vi "SECADO_JKI_v120.vi"() -> ()   [LabVIEW 2017] (continued)
C"=0.0, "P116.temperatura, C"=0.0, "P116.output, %"=0.0, "P116.output, W"=0.0, "Q.set.caudal, g/s"=0.0, "Q.caudal, g/s"=0.0, "Agua.evapor, g/s"=0.0, "Humedad.lecho, f1"=0.0, "Q.aire.seco, W"=0.0, "Q.evaporacion, W"=0.0, "Porosidad, "=0.0, "Vel.air.reactor, m/s"=0.0, "Temp.termopar.7, C"=0.0, "Temp.termopar.8, C"=0.0, "Temp.termopar.9, C"=0.0, "Presion.abs.ext, Pa"=0.0}, {"Tiempo (min)"=0.0, "Temperatura.ext, C"=0.0, "Humedad.Rel.ext, f1"=0.0, "Temp.pt100.1, C"=0.0, "Temp.pt100.2, C"=0.0, "Temp.pt100.3, C"=0.0, "Temp.pt100.4, C"=0.0, "Temp.termopar.5, C"=0.0, "Temp.termopar.6, C"=0.0, "Humedad.rel.3, f1"=0.0, "Humedad.rel.4, f1"=0.0, "Q.caudal.vol, m3/h"=0.0, "P116.set.temp, C"=0.0, "P116.temperatura, C"=0.0, "P116.output, %"=0.0, "P116.output, W"=0.0, "Q.set.caudal, g/s"=0.0, "Q.caudal, g/s"=0.0, "Agua.evapor, g/s"=0.0, "Humedad.lecho, f1"=0.0, "Q.aire.seco, W"=0.0, "Q.evaporacion, W"=0.0, "Porosidad, "=0.0, "Vel.air.reactor, m/s"=0.0, "Temp.termopar.7, C"=0.0, "Temp.termopar.8, C"=0.0, "Temp.termopar.9, C"=0.0, "Presion.abs.ext, Pa"=0.0}, {"Tiempo (min)"=0.0, "Temperatura.ext, C"=0.0, "Humedad.Rel.ext, f1"=0.0, "Temp.pt100.1, C"=0.0, "Temp.pt100.2, C"=0.0, "Temp.pt100.3, C"=0.0, "Temp.pt100.4, C"=0.0, "Temp.termopar.5, C"=0.0, "Temp.termopar.6, C"=0.0, "Humedad.rel.3, f1"=0.0, "Humedad.rel.4, f1"=0.0, "Q.caudal.vol, m3/h"=0.0, "P116.set.temp, C"=0.0, "P116.temperatura, C"=0.0, "P116.output, %"=0.0, "P116.output, W"=0.0, "Q.set.caudal, g/s"=0.0, "Q.caudal, g/s"=0.0, "Agua.evapor, g/s"=0.0, "Humedad.lecho, f1"=0.0, "Q.aire.seco, W"=0.0, "Q.evaporacion, W"=0.0, "Porosidad, "=0.0, "Vel.air.reactor, m/s"=0.0, "Temp.termopar.7, C"=0.0, "Temp.termopar.8, C"=0.0, "Temp.termopar.9, C"=0.0, "Presion.abs.ext, Pa"=0.0}, {"Tiempo (min)"=0.0, "Temperatura.ext, C"=0.0, "Humedad.Rel.ext, f1"=0.0, "Temp.pt100.1, C"=0.0, "Temp.pt100.2, C"=0.0, "Temp.pt100.3, C"=0.0, "Temp.pt100.4, C"=0.0, "Temp.termopar.5, C"=0.0, "Temp.termopar.6, C"=0.0, "Humedad.rel.3, f1"=0.0, "Humedad.rel.4, f1"=0.0, "Q.caudal.vol, m3/h"=0.0, "P116.set.temp, C"=0.0, "P116.temperatura, C"=0.0, "P116.output, %"=0.0, "P116.output, W"=0.0, "Q.set.caudal, g/s"=0.0, "Q.caudal, g/s"=0.0, "Agua.evapor, g/s"=0.0, "Humedad.lecho, f1"=0.0, "Q.aire.seco, W"=0.0, "Q.evaporacion, W"=0.0, "Porosidad, "=0.0, "Vel.air.reactor, m/s"=0.0, "Temp.termopar.7, C"=0.0, "Temp.termopar.8, C"=0.0, "Temp.termopar.9, C"=0.0, "Presion.abs.ext, Pa"=0.0}, {"Tiempo (min)"=0.0, "Temperatura.ext, C"=0.0, "Humedad.Rel.ext, f1"=0.0, "Temp.pt100.1, C"=0.0, "Temp.pt100.2, C"=0.0, "Temp.pt100.3, C"=0.0, "Temp.pt100.4, C"=0.0, "Temp.termopar.5, C"=0.0, "Temp.termopar.6, C"=0.0, "Humedad.rel.3, f1"=0.0, "Humedad.rel.4, f1"=0.0, "Q.caudal.vol, m3/h"=0.0, "P116.set.temp, C"=0.0, "P116.temperatura, C"=0.0, "P116.output, %"=0.0, "P116.output, W"=0.0, "Q.set.caudal, g/s"=0.0, "Q.caudal, g/s"=0.0, "Agua.evapor, g/s"=0.0, "Humedad.lecho, f1"=0.0, "Q.aire.seco, W"=0.0, "Q.evaporacion, W"=0.0, "Porosidad, "=0.0, "Vel.air.reactor, m/s"=0.0, "Temp.termopar.7, C"=0.0, "Temp.termopar.8, C"=0.0, "Temp.termopar.9, C"=0.0, "Presion.abs.ext, Pa"=0.0}, {"Tiempo (min)"=0.0, "Temperatura.ext, C"=0.0, "Humedad.Rel.ext, f1"=0.0, "Temp.pt100.1, C"=0.0, "Temp.pt100.2, C"=0.0, "Temp.pt100.3, C"=0.0, "Temp.pt100.4, C"=0.0, "Temp.termopar.5, C"=0.0, "Temp.termopar.6, C"=0.0, "Humedad.rel.3, f1"=0.0, "Humedad.rel.4, f1"=0.0, "Q.caudal.vol, m3/h"=0.0, "P116.set.temp, C"=0.0, "P116.temperatura, C"=0.0, "P116.output, %"=0.0, "P116.output, W"=0.0, "Q.set.caudal, g/s"=0.0, "Q.caudal, g/s"=0.0, "Agua.evapor, g/s"=0.0, "Humedad.lecho, f1"=0.0, "Q.aire.seco, W"=0.0, "Q.evaporacion, W"=0.0, "Porosidad, "=0.0, "Vel.air.reactor, m/s"=0.0, "Temp.termopar.7, C"=0.0, "Temp.termopar.8, C"=0.0, "Temp.termopar.9, C"=0.0, "Presion.abs.ext, Pa"=0.0}, {"Tiempo (min)"=0.0, "Temperatura.ext, C"=0.0, "Humedad.Rel.ext, f1"=0.0, "Temp.pt100.1, C"=0.0, "Temp.pt100.2, C"=0.0, "Temp.pt100.3, C"=0.0, "Temp.pt100.4, C"=0.0, "Temp.termopar.5, C"=0.0, "Temp.termopar.6, C"=0.0, "Humedad.rel.3, f1"=0.0, "Humedad.rel.4, f1"=0.0, "Q.caudal.vol, m3/h"=0.0, "P116.set.temp, C"=0.0, "P116.temperatura, C"=0.0, "P116.output, %"=0.0, "P116.output, W"=0.0, "Q.set.caudal, g/s"=0.0, "Q.caudal, g/s"=0.0, "Agua.evapor, g/s"=0.0, "Humedad.lecho, f1"=0.0, "Q.aire.seco, W"=0.0, "Q.evaporacion, W"=0.0, "Porosidad, "=0.0, "Vel.air.reactor, m/s"=0.0, "Temp.termopar.7, C"=0.0, "Temp.termopar.8, C"=0.0, "Temp.termopar.9, C"=0.0, "Presion.abs.ext, Pa"=0.0}, {"Tiempo (min)"=0.0, "Temperatura.ext, C"=0.0, "Humedad.Rel.ext, f1"=0.0, "Temp.pt100.1, C"=0.0, "Temp.pt100.2, C"=0.0, "Temp.pt100.3, C"=0.0, "Temp.pt100.4, C"=0.0, "Temp.termopar.5, C"=0.0, "Temp.termopar.6, C"=0.0, "Humedad.rel.3, f1"=0.0, "Humedad.rel.4, f1"=0.0, "Q.caudal.vol, m3/h"=0.0, "P116.set.temp, C"=0.0, "P116.temperatura, C"=0.0, "P116.output, %"=0.0, "P116.output, W"=0.0, "Q.set.caudal, g/s"=0.0, "Q.caudal, g/s"=0.0, "Agua.evapor, g/s"=0.0, "Humedad.lecho, f1"=0.0, "Q.aire.seco, W"=0.0, "Q.evaporacion, W"=0.0, "Porosidad, "=0.0, "Vel.air.reactor, m/s"=0.0, "Temp.termopar.7, C"=0.0, "Temp.termopar.8, C"=0.0, "Temp.termopar.9, C"=0.0, "Presion.abs.ext, Pa"=0.0}, {"Tiempo (min)"=0.0, "Temperatura.ext, C"=0.0, "Humedad.Rel.ext, f1"=0.0, "Temp.pt100.1, C"=0.0, "Temp.pt100.2, C"=0.0, "Temp.pt100.3, C"=0.0, "Temp.pt100.4, C"=0.0, "Temp.termopar.5, C"=0.0, "Temp.termopar.6, C"=0.0, "Humedad.rel.3, f1"=0.0, "Humedad.rel.4, f1"=0.0, "Q.caudal.vol, m3/h"=0.0, "P116.set.temp, C"=0.0, "P116.temperatura, C"=0.0, "P116.output, %"=0.0, "P116.output, W"=0.0, "Q.set.caudal, g/s"=0.0, "Q.caudal, g/s"=0.0, "Agua.evapor, g/s"=0.0, "Humedad.lecho, f1"=0.0, "Q.aire.seco, W"=0.0, "Q.evaporacion, W"=0.0, "Porosidad, "=0.0, "Vel.air.reactor, m/s"=0.0, "Temp.termopar.7, C"=0.0, "Temp.termopar.8, C"=0.0, "Temp.termopar.9, C"=0.0, "Presion.abs.ext, Pa"=0.0}, {"Tiempo (min)"=0.0, "Temperatura.ext, C"=0.0, "Humedad.Rel.ext, f1"=0.0, "Temp.pt100.1, C"=0.0, "Temp.pt100.2, C"=0.0, "Temp.pt100.3, C"=0.0, "Temp.pt100.4, C"=0.0, "Temp.termopar.5, C"=0.0, "Temp.termopar.6, C"=0.0, "Humedad.rel.3, f1"=0.0, "Humedad.rel.4, f1"=0.0, "Q.caudal.vol, m3/h"=0.0, "P116.set.temp, C"=0.0, "P116.temperatura, C"=0.0, "P116.output, %"=0.0, "P116.output, W"=0.0, "Q.set.caudal, g/s"=0.0, "Q.caudal, g/s"=0.0, "Agua.evapor, g/s"=0.0, "Humedad.lecho, f1"=0.0, "Q.aire.seco, W"=0.0, "Q.evaporacion, W"=0.0, "Porosidad, "=0.0, "Vel.air.reactor, m/s"=0.0, "Temp.termopar.7, C"=0.0, "Temp.termopar.8, C"=0.0, "Temp.termopar.9, C"=0.0, "Presion.abs.ext, Pa"=0.0}, {"Tiempo (min)"=0.0, "Temperatura.ext, C"=0.0, "Humedad.Rel.ext, f1"=0.0, "Temp.pt100.1, C"=0.0, "Temp.pt100.2, C"=0.0, "Temp.pt100.3, C"=0.0, "Temp.pt100.4, C"=0.0, "Temp.termopar.5, C"=0.0, "Temp.termopar.6, C"=0.0, "Humedad.rel.3, f1"=0.0, "Humedad.rel.4, f1"=0.0, "Q.caudal.vol, m3/h"=0.0, "P116.set.temp, C"=0.0, "P116.temperatura, C"=0.0, "P116.output, %"=0.0, "P116.output, W"=0.0, "Q.set.caudal, g/s"=0.0, "Q.caudal, g/s"=0.0, "Agua.evapor, g/s"=0.0, "Humedad.lecho, f1"=0.0, "Q.aire.seco, W"=0.0, "Q.evaporacion, W"=0.0, "Porosidad, "=0.0, "Vel.air.reactor, m/s"=0.0, "Temp.termopar.7, C"=0.0, "Temp.termopar.8, C"=0.0, "Temp.termopar.9, C"=0.0, "Presion.abs.ext, Pa"=0.0}, {"Tiempo (min)"=0.0, "Temperatura.ext, C"=0.0, "Humedad.Rel.ext, f1"=0.0, "Temp.pt100.1, C"=0.0, "Temp.pt100.2, C"=0.0, "Temp.pt100.3, C"=0.0, "Temp.pt100.4, C"=0.0, "Temp.termopar.5, C"=0.0, "Temp.termopar.6, C"=0.0, "Humedad.rel.3, f1"=0.0, "Humedad.rel.4, f1"=0.0, "Q.caudal.vol, m3/h"=0.0, "P116.set.temp, C"=0.0, "P116.temperatura, C"=0.0, "P116.output, %"=0.0, "P116.output, W"=0.0, "Q.set.caudal, g/s"=0.0, "Q.caudal, g/s"=0.0, "Agua.evapor, g/s"=0.0, "Humedad.lecho, f1"=0.0, "Q.aire.seco, W"=0.0, "Q.evaporacion, W"=0.0, "Porosidad, "=0.0, "Vel.air.reactor, m/s"=0.0, "Temp.termopar.7, C"=0.0, "Temp.termopar.8, C"=0.0, "Temp.termopar.9, C"=0.0, "Presion.abs.ext, Pa"=0.0}, {"Tiempo (min)"=0.0, "Temperatura.ext, C"=0.0, "Humedad.Rel.ext, f1"=0.0, "Temp.pt100.1, C"=0.0, "Temp.pt100.2, C"=0.0, "Temp.pt100.3, C"=0.0, "Temp.pt100.4, C"=0.0, "Temp.termopar.5, C"=0.0, "Temp.termopar.6, C"=0.0, "Humedad.rel.3, f1"=0.0, "Humedad.rel.4, f1"=0.0, "Q.caudal.vol, m3/h"=0.0, "P116.set.temp, C"=0.0, "P116.temperatura, C"=0.0, "P116.output, %"=0.0, "P116.output, W"=0.0, "Q.set.caudal, g/s"=0.0, "Q.caudal, g/s"=0.0, "Agua.evapor, g/s"=0.0, "Humedad.lecho, f1"=0.0, "Q.aire.seco, W"=0.0, "Q.evaporacion, W"=0.0, "Porosidad, "=0.0, "Vel.air.reactor, m/s"=0.0, "Temp.termopar.7, C"=0.0, "Temp.termopar.8, C"=0.0, "Temp.termopar.9, C"=0.0, "Presion.abs.ext, Pa"=0.0}, {"Tiempo (min)"=0.0, "Temperatura.ext, C"=0.0, "Humedad.Rel.ext, f1"=0.0, "Temp.pt100.1, C"=0.0, "Temp.pt100.2, C"=0.0, "Temp.pt100.3, C"=0.0, "Temp.pt100.4, C"=0.0, "Temp.termopar.5, C"=0.0, "Temp.termopar.6, C"=0.0, "Humedad.rel.3, f1"=0.0, "Humedad.rel.4, f1"=0.0, "Q.caudal.vol, m3/h"=0.0, "P116.set.temp, C"=0.0, "P116.temperatura, C"=0.0, "P116.output, %"=0.0, "P116.output, W"=0.0, "Q.set.caudal, g/s"=0.0, "Q.caudal, g/s"=0.0, "Agua.evapor, g/s"=0.0, "Humedad.lecho, f1"=0.0, "Q.aire.seco, W"=0.0, "Q.evaporacion, W"=0.0, "Porosidad, "=0.0, "Vel.air.reactor, m/s"=0.0, "Temp.termopar.7, C"=0.0, "Temp.termopar.8, C"=0.0, "Temp.termopar.9, C"=0.0, "Presion.abs.ext, Pa"=0.0}, {"Tiempo (min)"=0.0, "Temperatura.ext, C"=0.0, "Humedad.Rel.ext, f1"=0.0, "Temp.pt100.1, C"=0.0, "Temp.pt100.2, C"=0.0, "Temp.pt100.3, C"=0.0, "Temp.pt100.4, C"=0.0, "Temp.termopar.5, C"=0.0, "Temp.termopar.6, C"=0.0, "Humedad.rel.3, f1"=0.0, "Humedad.rel.4, f1"=0.0, "Q.caudal.vol, m3/h"=0.0, "P116.set.temp, C"=0.0, "P116.temperatura, C"=0.0, "P116.output, %"=0.0, "P116.output, W"=0.0, "Q.set.caudal, g/s"=0.0, "Q.caudal, g/s"=0.0, "Agua.evapor, g/s"=0.0, "Humedad.lecho, f1"=0.0, "Q.aire.seco, W"=0.0, "Q.evaporacion, W"=0.0, "Porosidad, "=0.0, "Vel.air.reactor, m/s"=0.0, "Temp.termopar.7, C"=0.0, "Temp.termopar.8, C"=0.0, "Temp.termopar.9, C"=0.0, "Presion.abs.ext, Pa"=0.0}, {"Tiempo (min)"=0.0, "Temperatura.ext, C"=0.0, "Humedad.Rel.ext, f1"=0.0, "Temp.pt100.1, C"=0.0, "Temp.pt100.2, C"=0.0, "Temp.pt100.3, C"=0.0, "Temp.pt100.4, C"=0.0, "Temp.termopar.5, C"=0.0, "Temp.termopar.6, C"=0.0, "Humedad.rel.3, f1"=0.0, "Humedad.rel.4, f1"=0.0, "Q.caudal.vol, m3/h"=0.0, "P116.set.temp, C"=0.0, "P116.temperatura, C"=0.0, "P116.output, %"=0.0, "P116.output, W"=0.0, "Q.set.caudal, g/s"=0.0, "Q.caudal, g/s"=0.0, "Agua.evapor, g/s"=0.0, "Humedad.lecho, f1"=0.0, "Q.aire.seco, W"=0.0, "Q.evaporacion, W"=0.0, "Porosidad, "=0.0, "Vel.air.reactor, m/s"=0.0, "Temp.termopar.7, C"=0.0, "Temp.termopar.8, C"=0.0, "Temp.termopar.9, C"=0.0, "Presion.abs.ext, Pa"=0.0}, {"Tiempo (min)"=0.0, "Temperatura.ext, C"=0.0, "Humedad.Rel.ext, f1"=0.0, "Temp.pt100.1, C"=0.0, "Temp.pt100.2, C"=0.0, "Temp.pt100.3, C"=0.0, "Temp.pt100.4, C"=0.0, "Temp.termopar.5, C"=0.0, "Temp.termopar.6, C"=0.0, "Humedad.rel.3, f1"=0.0, "Humedad.rel.4, f1"=0.0, "Q.caudal.vol, m3/h"=0.0, "P116.set.temp, C"=0.0, "P116.temperatura, C"=0.0, "P116.output, %"=0.0, "P116.output, W"=0.0, "Q.set.caudal, g/s"=0.0, "Q.caudal, g/s"=0.0, "Agua.evapor, g/s"=0.0, "Humedad.lecho, f1"=0.0, "Q.aire.seco, W"=0.0, "Q.evaporacion, W"=0.0, "Porosidad, "=0.0, "Vel.air.reactor, m/s"=0.0, "Temp.termopar.7, C"=0.0, "Temp.termopar.8, C"=0.0, "Temp.termopar.9, C"=0.0, "Presion.abs.ext, Pa"=0.0}, {"Tiempo (min)"=0.0, "Temperatura.ext, C"=0.0, "Humedad.Rel.ext, f1"=0.0, "Temp.pt100.1, C"=0.0, "Temp.pt100.2, C"=0.0, "Temp.pt100.3, C"=0.0, "Temp.pt100.4, C"=0.0, "Temp.termopar.5, C"=0.0, "Temp.termopar.6, C"=0.0, "Humedad.rel.3, f1"=0.0, "Humedad.rel.4, f1"=0.0, "Q.caudal.vol, m3/h"=0.0, "P116.set.temp, C"=0.0, "P116.temperatura, C"=0.0, "P116.output, %"=0.0, "P116.output, W"=0.0, "Q.set.caudal, g/s"=0.0, "Q.caudal, g/s"=0.0, "Agua.evapor, g/s"=0.0, "Humedad.lecho, f1"=0.0, "Q.aire.seco, W"=0.0, "Q.evaporacion, W"=0.0, "Porosidad, "=0.0, "Vel.air.reactor, m/s"=0.0, "Temp.termopar.7, C"=0.0, "Temp.termopar.8, C"=0.0, "Temp.termopar.9, C"=0.0, "Presion.abs.ext, Pa"=0.0}, {"Tiempo (min)"=0.0, "Temperatura.ext, C"=0.0, "Humedad.Rel.ext, f1"=0.0, "Temp.pt100.1, C"=0.0, "Temp.pt100.2, C"=0.0, "Temp.pt100.3, C"=0.0, "Temp.pt100.4, C"=0.0, "Temp.termopar.5, C"=0.0, "Temp.termopar.6, C"=0.0, "Humedad.rel.3, f1"=0.0, "Humedad.rel.4, f1"=0.0, "Q.caudal.vol, m3/h"=0.0, "P116.set.temp, C"=0.0, "P116.temperatura, C"=0.0, "P116.output, %"=0.0, "P116.output, W"=0.0, "Q.set.caudal, g/s"=0.0, "Q.caudal, g/s"=0.0, "Agua.evapor, g/s"=0.0, "Humedad.lecho, f1"=0.0, "Q.aire.seco, W"=0.0, "Q.evaporacion, W"=0.0, "Porosidad, "=0.0, "Vel.air.reactor, m/s"=0.0, "Temp.termopar.7, C"=0.0, "Temp.termopar.8, C"=0.0, "Temp.termopar.9, C"=0.0, "Presion.abs.ext, Pa"=0.0}, {"Tiempo (min)"=0.0, "Temperatura.ext, C"=0.0, "Humedad.Rel.ext, f1"=0.0, "Temp.pt100.1, C"=0.0, "Temp.pt100.2, C"=0.0, "Temp.pt100.3, C"=0.0, "Temp.pt100.4, C"=0.0, "Temp.termopar.5, C"=0.0, "Temp.termopar.6, C"=0.0, "Humedad.rel.3, f1"=0.0, "Humedad.rel.4, f1"=0.0, "Q.caudal.vol, m3/h"=0.0, "P116.set.temp, C"=0.0, "P116.temperatura, C"=0.0, "P116.output, %"=0.0, "P116.output, W"=0.0, "Q.set.caudal, g/s"=0.0, "Q.caudal, g/s"=0.0, "Agua.evapor, g/s"=0.0, "Humedad.lecho, f1"=0.0, "Q.aire.seco, W"=0.0, "Q.evaporacion, W"=0.0, "Porosidad, "=0.0, "Vel.air.reactor, m/s"=0.0, "Temp.termopar.7, C"=0.0, "Temp.termopar.8, C"=0.0, "Temp.termopar.9, C"=0.0, "Presion.abs.ext, Pa"=0.0}, {"Tiempo (min)"=0.0, "Temperatura.ext, C"=0.0, "Humedad.Rel.ext, f1"=0.0, "Temp.pt100.1, C"=0.0, "Temp.pt100.2, C"=0.0, "Temp.pt100.3, C"=0.0, "Temp.pt100.4, C"=0.0, "Temp.termopar.5, C"=0.0, "Temp.termopar.6, C"=0.0, "Humedad.rel.3, f1"=0.0, "Humedad.rel.4, f1"=0.0, "Q.caudal.vol, m3/h"=0.0, "P116.set.temp, C"=0.0, "P116.temperatura, C"=0.0, "P116.output, %"=0.0, "P116.output, W"=0.0, "Q.set.caudal, g/s"=0.0, "Q.caudal, g/s"=0.0, "Agua.evapor, g/s"=0.0, "Humedad.lecho, f1"=0.0, "Q.aire.seco, W"=0.0, "Q.evaporacion, W"=0.0, "Porosidad, "=0.0, "Vel.air.reactor, m/s"=0.0, "Temp.termopar.7, C"=0.0, "Temp.termopar.8, C"=0.0, "Temp.termopar.9, C"=0.0, "Presion.abs.ext, Pa"=0.0}, {"Tiempo (min)"=0.0, "Temperatura.ext, C"=0.0, "Humedad.Rel.ext, f1"=0.0, "Temp.pt100.1, C"=0.0, "Temp.pt100.2, C"=0.0, "Temp.pt100.3, C"=0.0, "Temp.pt100.4, C"=0.0, "Temp.termopar.5, C"=0.0, "Temp.termopar.6, C"=0.0, "Humedad.rel.3, f1"=0.0, "Humedad.rel.4, f1"=0.0, "Q.caudal.vol, m3/h"=0.0, "P116.set.temp, C"=0.0, "P116.temperatura, C"=0.0, "P116.output, %"=0.0, "P116.output, W"=0.0, "Q.set.caudal, g/s"=0.0, "Q.caudal, g/s"=0.0, "Agua.evapor, g/s"=0.0, "Humedad.lecho, f1"=0.0, "Q.aire.seco, W"=0.0, "Q.evaporacion, W"=0.0, "Porosidad, "=0.0, "Vel.air.reactor, m/s"=0.0, "Temp.termopar.7, C"=0.0, "Temp.termopar.8, C"=0.0, "Temp.termopar.9, C"=0.0, "Presion.abs.ext, Pa"=0.0}, {"Tiempo (min)"=0.0, "Temperatura.ext, C"=0.0, "Humedad.Rel.ext, f1"=0.0, "Temp.pt100.1, C"=0.0, "Temp.pt100.2, C"=0.0, "Temp.pt100.3, C"=0.0, "Temp.pt100.4, C"=0.0, "Temp.termopar.5, C"=0.0, "Temp.termopar.6, C"=0.0, "Humedad.rel.3, f1"=0.0, "Humedad.rel.4, f1"=0.0, "Q.caudal.vol, m3/h"=0.0, "P116.set.temp, C"=0.0, "P116.temperatura, C"=0.0, "P116.output, %"=0.0, "P116.output, W"=0.0, "Q.set.caudal, g/s"=0.0, "Q.caudal, g/s"=0.0, "Agua.evapor, g/s"=0.0, "Humedad.lecho, f1"=0.0, "Q.aire.seco, W"=0.0, "Q.evaporacion, W"=0.0, "Porosidad, "=0.0, "Vel.air.reactor, m/s"=0.0, "Temp.termopar.7, C"=0.0, "Temp.termopar.8, C"=0.0, "Temp.termopar.9, C"=0.0, "Presion.abs.ext, Pa"=0.0}, {"Tiempo (min)"=0.0, "Temperatura.ext, C"=0.0, "Humedad.Rel.ext, f1"=0.0, "Temp.pt100.1, C"=0.0, "Temp.pt100.2, C"=0.0, "Temp.pt100.3, C"=0.0, "Temp.pt100.4, C"=0.0, "Temp.termopar.5, C"=0.0, "Temp.termopar.6, C"=0.0, "Humedad.rel.3, f1"=0.0, "Humedad.rel.4, f1"=0.0, "Q.caudal.vol, m3/h"=0.0, "P116.set.temp, C"=0.0, "P116.temperatura, C"=0.0, "P116.output, %"=0.0, "P116.output, W"=0.0, "Q.set.caudal, g/s"=0.0, "Q.caudal, g/s"=0.0, "Agua.evapor, g/s"=0.0, "Humedad.lecho, f1"=0.0, "Q.aire.seco, W"=0.0, "Q.evaporacion, W"=0.0, "Porosidad, "=0.0, "Vel.air.reactor, m/s"=0.0, "Temp.termopar.7, C"=0.0, "Temp.termopar.8, C"=0.0, "Temp.termopar.9, C"=0.0, "Presion.abs.ext, Pa"=0.0}, {"Tiempo (min)"=0.0, "Temperatura.ext, C"=0.0, "Humedad.Rel.ext, f1"=0.0, "Temp.pt100.1, C"=0.0, "Temp.pt100.2, C"=0.0, "Temp.pt100.3, C"=0.0, "Temp.pt100.4, C"=0.0, "Temp.termopar.5, C"=0.0, "Temp.termopar.6, C"=0.0, "Humedad.rel.3, f1"=0.0, "Humedad.rel.4, f1"=0.0, "Q.caudal.vol, m3/h"=0.0, "P116.set.temp, C"=0.0, "P116.temperatura, C"=0.0, "P116.output, %"=0.0, "P116.output, W"=0.0, "Q.set.caudal, g/s"=0.0, "Q.caudal, g/s"=0.0, "Agua.evapor, g/s"=0.0, "Humedad.lecho, f1"=0.0, "Q.aire.seco, W"=0.0, "Q.evaporacion, W"=0.0, "Porosidad, "=0.0, "Vel.air.reactor, m/s"=0.0, "Temp.termopar.7, C"=0.0, "Temp.termopar.8, C"=0.0, "Temp.termopar.9, C"=0.0, "Presion.abs.ext, Pa"=0.0}, {"Tiempo (min)"=0.0, "Temperatura.ext, C"=0.0, "Humedad.Rel.ext, f1"=0.0, "Temp.pt100.1, C"=0.0, "Temp.pt100.2, C"=0.0, "Temp.pt100.3, C"=0.0, "Temp.pt100.4, C"=0.0, "Temp.termopar.5, C"=0.0, "Temp.termopar.6, C"=0.0, "Humedad.rel.3, f1"=0.0, "Humedad.rel.4, f1"=0.0, "Q.caudal.vol, m3/h"=0.0, "P116.set.temp, C"=0.0, "P116.temperatura, C"=0.0, "P116.output, %"=0.0, "P116.output, W"=0.0, "Q.set.caudal, g/s"=0.0, "Q.caudal, g/s"=0.0, "Agua.evapor, g/s"=0.0, "Humedad.lecho, f1"=0.0, "Q.aire.seco, W"=0.0, "Q.evaporacion, W"=0.0, "Porosidad, "=0.0, "Vel.air.reactor, m/s"=0.0, "Temp.termopar.7, C"=0.0, "Temp.termopar.8, C"=0.0, "Temp.termopar.9, C"=0.0, "Presion.abs.ext, Pa"=0.0}, {"Tiempo (min)"=0.0, "Temperatura.ext, C"=0.0, "Humedad.Rel.ext, f1"=0.0, "Temp.pt100.1, C"=0.0, "Temp.pt100.2, C"=0.0, "Temp.pt100.3, C"=0.0, "Temp.pt100.4, C"=0.0, "Temp.termopar.5, C"=0.0, "Temp.termopar.6, C"=0.0, "Humedad.rel.3, f1"=0.0, "Humedad.rel.4, f1"=0.0, "Q.caudal.vol, m3/h"=0.0, "P116.set.temp, C"=0.0, "P116.temperatura, C"=0.0, "P116.output, %"=0.0, "P116.output, W"=0.0, "Q.set.caudal, g/s"=0.0, "Q.caudal, g/s"=0.0, "Agua.evapor, g/s"=0.0, "Humedad.lecho, f1"=0.0, "Q.aire.seco, W"=0.0, "Q.evaporacion, W"=0.0, "Porosidad, "=0.0, "Vel.air.reactor, m/s"=0.0, "Temp.termopar.7, C"=0.0, "Temp.termopar.8, C"=0.0, "Temp.termopar.9, C"=0.0, "Presion.abs.ext, Pa"=0.0}, {"Tiempo (min)"=0.0, "Temperatura.ext, C"=0.0, "Humedad.Rel.ext, f1"=0.0, "Temp.pt100.1, C"=0.0, "Temp.pt100.2, C"=0.0, "Temp.pt100.3, C"=0.0, "Temp.pt100.4, C"=0.0, "Temp.termopar.5, C"=0.0, "Temp.termopar.6, C"=0.0, "Humedad.rel.3, f1"=0.0, "Humedad.rel.4, f1"=0.0, "Q.caudal.vol, m3/h"=0.0, "P116.set.temp, C"=0.0, "P116.temperatura, C"=0.0, "P116.output, %"=0.0, "P116.output, W"=0.0, "Q.set.caudal, g/s"=0.0, "Q.caudal, g/s"=0.0, "Agua.evapor, g/s"=0.0, "Humedad.lecho, f1"=0.0, "Q.aire.seco, W"=0.0, "Q.evaporacion, W"=0.0, "Porosidad, "=0.0, "Vel.air.reactor, m/s"=0.0, "Temp.termopar.7, C"=0.0, "Temp.termopar.8, C"=0.0, "Temp.termopar.9, C"=0.0, "Presion.abs.ext, Pa"=0.0}]  # data array
        w122 = path "C:/Users/usuario/Documents/LabVIEW Data/testSecado.dat"  # Filename
        w125 = FALSE  # Step.timeout?
        w123 = ""  # Status string
        # "Número de datos maximo para graficar"
        # "Array de datos: rellenar constante con 3600 registros a 0"
        # "Initialize the shift-register data, here.\n(data names are defined by what you wire into the bundle function)"
        n39 = Bundle By Name(cluster=w132, "datos.Ensayo"=w129, "data array"=w130, "nPuntos"=w121, "Filename"=w122, "Status.string"=w123, "Step.sample.time"=w124, "Step.timeout?"=w125, "Prog.running?"=w126, "Prog.aborted?"=w127, "Seq.loaded?"=w128, "#Datos"=w120) -> (w131:T19)
        n40 = call <vilib>:"Add State(s) to Queue__JKI_lib_State_Machine.vi"("State(s) in (\"\")"=w135) -> ("States Out"=w134:string)  [unwired: 14 in]
      }
      frame "Data: Cleanup" {
        # "Cleanup any data and references, here.\n(this is called automatically, by the Macro: Exit)"
        n41 = Unbundle By Name(w136) -> ("Core.Current VI Reference"=w139:refnum<vi>)
        n42 = Close Reference(reference=w139, error in (no error)=w138) -> (error out=w137:errorcluster)
        n43 = call <vilib>:"Add State(s) to Queue__JKI_lib_State_Machine.vi"("State(s) in (\"\")"=w141) -> ("States Out"=w140:string)  [unwired: 14 in]
      }
      frame "---------- Instruments ----------" {
        # "Do not put any code in this frame.\n(It is a separator no-op. You can make a copy of this frame to create a new Data frame)"
        n44 = call <vilib>:"Add State(s) to Queue__JKI_lib_State_Machine.vi"("State(s) in (\"\")"=w145) -> ("States Out"=w144:string)  [unwired: 14 in]
      }
      frame "Instruments: Serial Comms" {
        # "Your code here.\n(You can make a copy of, or modify, this frame)"
        n45 = call "SECADO_enterComms.vi"("error in (no error)"=w149) -> ("error out"=w148:errorcluster, "Comunicaciones"=w146:T9)  [unwired: 8 in, 1 out]
        n46 = Bundle By Name(cluster=w150, "Comunicaciones"=w146) -> (w147:T19)
        n47 = call <vilib>:"Add State(s) to Queue__JKI_lib_State_Machine.vi"("State(s) in (\"\")"=w152) -> ("States Out"=w151:string)  [unwired: 14 in]
      }
      frame "Instruments: Agilent Initialize" {
        # "Read Agilent channels\n(only for information)"
        # "Your code here.\n(You can make a copy of, or modify, this frame)"
        n48 = Unbundle By Name(w159) -> ("Comunicaciones.AGL"=w157:bool, "Comunicaciones.Agilent"=w158:refnum<visa-resource-name>)
        n49 = call "Agilent ReadConfigFile.vi"("Error In"=w154) -> ("Error Out"=w153:errorcluster, "Dispositivos"=→"Dispositivos":T3, "configuration file path"=→"Agilent.configuracion.file":path)  [unwired: 7 in]
        n50 = call "34970_Module.vi"("Agilent 34970A"=w157, "Command"=34970_Module_Control."INICIALIZA", "error in (no error)"=w153, "VISA Agilent 34970A"=w158) -> ("error out"=w160:errorcluster)  [unwired: 3 in, 4 out]
        n51 = call <vilib>:"Add State(s) to Queue__JKI_lib_State_Machine.vi"("State(s) in (\"\")"=w163) -> ("States Out"=w162:string)  [unwired: 14 in]
      }
      frame "Instruments: Agilent Close" {
        # "Your code here.\n(You can make a copy of, or modify, this frame)"
        n52 = Unbundle By Name(w167) -> ("Comunicaciones.AGL"=w165:bool, "Comunicaciones.Agilent"=w166:refnum<visa-resource-name>)
        n53 = call "34970_Module.vi"("Agilent 34970A"=w165, "Command"=34970_Module_Control."SHUTDOWN", "error in (no error)"=w164, "VISA Agilent 34970A"=w166) -> ("error out"=w168:errorcluster)  [unwired: 3 in, 4 out]
        n54 = call <vilib>:"Add State(s) to Queue__JKI_lib_State_Machine.vi"("State(s) in (\"\")"=w171) -> ("States Out"=w170:string)  [unwired: 14 in]
      }
      frame "Instruments: Eurotherm Initialize" {
        # "Your code here.\n(Eurotherm se inicializa, lee (o programa) y cierra en la misma ventana)"
        # "Your code here.\n(You can make a copy of, or modify, this frame)"
        n55 = Unbundle By Name(w173) -> ()  [unwired: 3 out]
        n56 = call <vilib>:"Add State(s) to Queue__JKI_lib_State_Machine.vi"("State(s) in (\"\")"=w175) -> ("States Out"=w174:string)  [unwired: 14 in]
      }
      frame "Instruments: Eurotherm Close" {
        # "Your code here.\n(Eurotherm se inicializa, lee (o programa) y cierra en la misma ventana)"
        # "Your code here.\n(You can make a copy of, or modify, this frame)"
        n57 = Unbundle By Name(w177) -> ()  [unwired: 2 out]
        n58 = call <vilib>:"Add State(s) to Queue__JKI_lib_State_Machine.vi"("State(s) in (\"\")"=w179) -> ("States Out"=w178:string)  [unwired: 14 in]
      }
      frame "---------- Timing ----------" {
        # "Do not put any code in this frame.\n(It is a separator no-op. You can make a copy of this frame to create a new UI frame)"
        n59 = call <vilib>:"Add State(s) to Queue__JKI_lib_State_Machine.vi"("State(s) in (\"\")"=w183) -> ("States Out"=w182:string)  [unwired: 14 in]
      }
      frame "Timing: Initialize Total Time" {
        # "Initialize total time counter in minutes here.\n(data names are defined by what you wire into the bundle function)"
        n60 = call "elapsedTotalMinutesModule.vi"("Command"=Timing_Module_Control."Initialize Time", "error in (no error)"=w185) -> ("error out"=w184:errorcluster)  [unwired: 7 in, 2 out]
        n61 = call <vilib>:"Add State(s) to Queue__JKI_lib_State_Machine.vi"("State(s) in (\"\")"=w189) -> ("States Out"=w188:string)  [unwired: 14 in]
      }
      frame "Timing: Measure Total Time" {
        # "Initialize total time counter in minutes here.\n(data names are defined by what you wire into the bundle function)"
        n62 = call "elapsedTotalMinutesModule.vi"("Command"=Timing_Module_Control."Check Time", "error in (no error)"=w198) -> ("error out"=w197:errorcluster, "Elapsed Out"=w192:dbl)  [unwired: 7 in, 1 out]
        n63 = Unbundle By Name(w191) -> ("datos.Ensayo.Tiempo (min)"=w195:dbl)
        n64 = Subtract(x=w192, y=w195) -> (x-y=w194:dbl)
        n65 = Multiply(x=w194, y=60.0) -> (x*y=w190:dbl)
        "dt.ciclo, s" <- w190
        n66 = Bundle By Name(cluster=w191, "datos.Ensayo.Tiempo (min)"=w192, "delta.t.ciclo"=w190) -> (w196:T19)
        n67 = call <vilib>:"Add State(s) to Queue__JKI_lib_State_Machine.vi"("State(s) in (\"\")"=w201) -> ("States Out"=w200:string)  [unwired: 14 in]
      }
      frame "Timing: Initialize Sample Time" {
        # "Initialize sample time in seconds, used for next sample\n(data names are defined by what you wire into the bundle function)"
        n68 = call "elapsedSamplingSecondsModule.vi"("Command"=Timing_Module_Control."Initialize Time", "error in (no error)"=w206) -> ("error out"=w205:errorcluster)  [unwired: 7 in, 2 out]
        n69 = Bundle By Name(cluster=w207, "Step.timeout?"=FALSE ("Step Timeout?")) -> (w203:T19)
        n70 = call <vilib>:"Add State(s) to Queue__JKI_lib_State_Machine.vi"("State(s) in (\"\")"=w209) -> ("States Out"=w208:string)  [unwired: 14 in]
      }
      frame "Timing: Measure Sample Time" {
        # "Initialize total time counter in minutes here.\n(data names are defined by what you wire into the bundle function)"
        n71 = Multiply(x="t.muestreo, s", y=1.0 ("x")) -> (x*y=w215:dbl)
        n72 = call "elapsedSamplingSecondsModule.vi"("Command"=Timing_Module_Control."Check Time", "error in (no error)"=w218, "Time In"=w215) -> ("error out"=w217:errorcluster, "Elapsed Out"=w212:dbl, "Time Elapsed"=w213:bool)  [unwired: 6 in]
        "t.ciclo, s" <- w212
        n73 = Bundle By Name(cluster=w219, "Step.timeout?"=w213, "Step.sample.time"=w212) -> (w214:T19)
        n74 = call <vilib>:"Add State(s) to Queue__JKI_lib_State_Machine.vi"("State(s) in (\"\")"=w221) -> ("States Out"=w220:string)  [unwired: 14 in]
      }
      frame "---------- UI ----------" {
        # "Do not put any code in this frame.\n(It is a separator no-op. You can make a copy of this frame to create a new UI frame)"
        n75 = call <vilib>:"Add State(s) to Queue__JKI_lib_State_Machine.vi"("State(s) in (\"\")"=w225) -> ("States Out"=w224:string)  [unwired: 14 in]
      }
      frame "UI: Initialize" {
        # "Initialize the User Interface, here.\n(this is called automatically, by the Macro: Init)"
        n76 = call <vilib>:"Add State(s) to Queue__JKI_lib_State_Machine.vi"("State(s) in (\"\")"=w229) -> ("States Out"=w228:string)  [unwired: 14 in]
      }
      frame "UI: Cursor Set" {
        # "Argument"
        # "Set and Unset Cursor Busy.\n(Usage: \"UI: Cursor Set >> Busy|Idle\")"
        n77 = case shown="\"Idle\", Default" w230 {
          tunnel: w232 -> [w237 w239]
          tunnel: [w236 w238] -> w231
          frame "Idle", Default {
            n78 = call <vilib>:"Unset Busy.vi"("error in (no error)"=w237) -> ("error out"=w236:errorcluster)  [unwired: 10 in]
          }
          frame "Busy" {
            n79 = call <vilib>:"Set Busy.vi"("error in (no error)"=w239) -> ("error out"=w238:errorcluster)  [unwired: 9 in, 1 out]
          }
        }
        n80 = call <vilib>:"Add State(s) to Queue__JKI_lib_State_Machine.vi"("State(s) in (\"\")"=w235) -> ("States Out"=w234:string)  [unwired: 14 in]
      }
      frame "UI: Front Panel State" {
        # "Argument"
        # "Set Front Panel Open or Closed\n(Usage: \"UI: Front Panel State >> Open|Close\")"
        n81 = Unbundle By Name(w242) -> ("Core.Current VI Reference"=w241:refnum<vi>)
        n82 = case shown="\"Open\", \"Standard\", Default" w240 {
          tunnel: w244 -> [w252 w267 w278 w291 w304]
          tunnel: [w254 w268 w280 w293 w306] -> w243
          tunnel: w241 -> [w253 w265 w279 w292 w305]
          frame "Open", "Standard", Default {
            w247 = T7."Standard" ("State")
            n83 = property class="VI"(reference=w253, error in=w252) -> (reference out=w250:refnum<vi>, error out=w251:errorcluster, "FP.State"=w249:T7)
            n84 = Not Equal?(x=w249, y=w247) -> (x != y?=w248:bool)
            n85 = case shown="False" w248 {
              tunnel: [w258 w260] -> w254
              tunnel: w251 -> [w257 w260]
              tunnel: w250 -> [w256 _]
              tunnel: w247 -> [w255 _]
              frame True {
                n86 = invoke class="VI" method="FP.Open"(reference=w256, error in=w257, "Activate"=TRUE, "State"=w255) -> (error out=w258:errorcluster)  [unwired: 1 in, 4 out]
              }
              frame False {
              }
            }
          }
          frame "Close", "Closed" {
            n87 = property class="VI"(reference=w265, error in=w267) -> (reference out=w264:refnum<vi>, error out=w266:errorcluster, "FP.State"=w262:T7)
            n88 = Not Equal?(x=w262, y=T7."Closed" ("Front Panel Window:State")) -> (x != y?=w261:bool)
            n89 = case shown="True" w261 {
              tunnel: [w269 w272] -> w268
              tunnel: w266 -> [w269 w271]
              tunnel: w264 -> [_ w270]
              frame False {
              }
              frame True {
                n90 = invoke class="VI" method="FP.Close"(reference=w270, error in=w271) -> (error out=w272:errorcluster)  [unwired: 1 in, 2 out]
              }
            }
          }
          frame "Hidden", "Hide" {
            w273 = T7."Hidden" ("State")
            n91 = property class="VI"(reference=w279, error in=w278) -> (reference out=w276:refnum<vi>, error out=w277:errorcluster, "FP.State"=w275:T7)
            n92 = Not Equal?(x=w275, y=w273) -> (x != y?=w274:bool)
            n93 = case shown="True" w274 {
              tunnel: [w284 w285] -> w280
              tunnel: w277 -> [w283 w285]
              tunnel: w276 -> [w282 _]
              tunnel: w273 -> [w281 _]
              frame True {
                n94 = invoke class="VI" method="FP.Open"(reference=w282, error in=w283, "State"=w281) -> (error out=w284:errorcluster)  [unwired: 2 in, 4 out]
              }
              frame False {
              }
            }
          }
          frame "Minimize", "Minimized" {
            w286 = T7."Minimized" ("State")
            n95 = property class="VI"(reference=w292, error in=w291) -> (reference out=w289:refnum<vi>, error out=w290:errorcluster, "FP.State"=w288:T7)
            n96 = Not Equal?(x=w288, y=w286) -> (x != y?=w287:bool)
            n97 = case shown="True" w287 {
              tunnel: [w297 w298] -> w293
              tunnel: w290 -> [w296 w298]
              tunnel: w289 -> [w295 _]
              tunnel: w286 -> [w294 _]
              frame True {
                n98 = invoke class="VI" method="FP.Open"(reference=w295, error in=w296, "State"=w294) -> (error out=w297:errorcluster)  [unwired: 2 in, 4 out]
              }
              frame False {
              }
            }
          }
          frame "Maximize", "Maximized" {
            w299 = T7."Maximized" ("State")
            n99 = property class="VI"(reference=w305, error in=w304) -> (reference out=w302:refnum<vi>, error out=w303:errorcluster, "FP.State"=w301:T7)
            n100 = Not Equal?(x=w301, y=w299) -> (x != y?=w300:bool)
            n101 = case shown="True" w300 {
              tunnel: [w310 w311] -> w306
              tunnel: w303 -> [w309 w311]
              tunnel: w302 -> [w308 _]
              tunnel: w299 -> [w307 _]
              frame True {
                n102 = invoke class="VI" method="FP.Open"(reference=w308, error in=w309, "State"=w307) -> (error out=w310:errorcluster)  [unwired: 2 in, 4 out]
              }
              frame False {
              }
            }
          }
        }
        n103 = call <vilib>:"Add State(s) to Queue__JKI_lib_State_Machine.vi"("State(s) in (\"\")"=w246) -> ("States Out"=w245:string)  [unwired: 14 in]
      }
      frame "UI: Update Status" {
        # "Set Front Panel Open or Closed\n(Usage: \"UI: Front Panel State >> Open|Close\")"
        n104 = Unbundle By Name(w315) -> ("Status.string"=→"Status":string)
        n105 = Unbundle By Name(w315) -> ("Prog.running?"=→"Prog. Running?":bool, "Prog.aborted?"=→"Prog. Aborted?":bool, "Seq.loaded?"=→"Seq. Loaded?":bool)
        n106 = call <vilib>:"Add State(s) to Queue__JKI_lib_State_Machine.vi"("State(s) in (\"\")"=w319) -> ("States Out"=w318:string)  [unwired: 14 in]
      }
      frame "UI: Update Interlock" {
        # "Set Front Panel Open or Closed\n(Usage: \"UI: Front Panel State >> Open|Close\")"
        n107 = Unbundle By Name(w321) -> ("Prog.running?"=w322:bool)
        n108 = case shown="True" w322 {
          tunnel: [w330 w332] -> w323
          tunnel: [w331 w333] -> w324
          tunnel: T13."Disabled and Grayed Out" ("Disabled") -> [w330 w333]
          tunnel: T13."Enabled" ("Disabled") -> [w331 w332]
          tunnel: [w331 w333] -> w320
          frame False {
            # "Si Prog. Running? FALSE --> \n\nEnable but.inicioMedida\nEnable but.Fin\nDisable but.finalMedida"
          }
          frame True {
            # "Si Prog. Running? TRUE -->\n \nDisable but.inicioMedida\nDisable but.Fin\nEnable but.finalMedida"
          }
        }
        n109 = property on="but.inicioMedida" class="Bool"("DisabledEnum"=w324) -> ()  [unwired: 2 in, 2 out]
        n110 = property on="but.finalMedida" class="Bool"("DisabledEnum"=w323) -> ()  [unwired: 2 in, 2 out]
        n111 = property on="but.Fin" class="Bool"("DisabledEnum"=w320) -> ()  [unwired: 2 in, 2 out]
        n112 = call <vilib>:"Add State(s) to Queue__JKI_lib_State_Machine.vi"("State(s) in (\"\")"=w329) -> ("States Out"=w328:string)  [unwired: 14 in]
      }
      frame "UI: Update Meas Data" {
        # "Set Front Panel Open or Closed\n(Usage: \"UI: Front Panel State >> Open|Close\")"
        n113 = Unbundle By Name(w342) -> ("datos.Ensayo"=→"Datos.ensayo":T4, "datos.Ensayo.Tiempo (min)"=→"t.ensayo, min":dbl, "datos.Ensayo.Temp.pt100.1, C"=→"TEMP_1, C":dbl, "datos.Ensayo.Temp.pt100.2, C"=→"TEMP_2, C":dbl, "datos.Ensayo.Temp.pt100.3, C"=→"TEMP_3, C":dbl, "datos.Ensayo.Temp.pt100.4, C"=→"TEMP_4, C":dbl, "datos.Ensayo.Humedad.rel.3, f1"=→"HUM_REL_3, f1":dbl, "datos.Ensayo.Humedad.rel.4, f1"=→"HUM_REL_4, f1":dbl, "datos.Ensayo.Q.caudal.vol, m3/h"=→"CAUDAL.vol, m³/h":dbl, "datos.Ensayo.P116.set.temp, C"=→"SET_TEMP_R, C":dbl, "datos.Ensayo.P116.temperatura, C"=→"TEMP_R, C":dbl, "datos.Ensayo.P116.output, W"=→"POTENCIA, W":dbl, "datos.Ensayo.Q.caudal, g/s"=→"CAUDAL, kg/h":dbl, "datos.Ensayo.Temperatura.ext, C"=→"TEMP_EXT, C":dbl, "datos.Ensayo.Temp.termopar.5, C"=→"TEMP_5, C":dbl, "datos.Ensayo.Temp.termopar.6, C"=→"TEMP_6, C":dbl, "Constantes.Ensayo.Hum_ext, f1"=→"HUM_EXT, f1":dbl, "Constantes.Ensayo.SET Caudal_vent, g/s"=→"SET_CAUDAL, g/s":dbl, "datos.Ensayo.Temp.termopar.7, C"=→"TEMP_7, C":dbl, "datos.Ensayo.Temp.termopar.8, C"=→"TEMP_8, C":dbl, "datos.Ensayo.Temp.termopar.9, C"=→"TEMP_9, C":dbl)  [unwired: 1 out]
        n114 = call <vilib>:"Add State(s) to Queue__JKI_lib_State_Machine.vi"("State(s) in (\"\")"=w358) -> ("States Out"=w357:string)  [unwired: 14 in]
      }
      frame "UI: Update Graphics" {
        # "Update Front Panel Graphics\n(Usage: \"UI: Front Panel State >> Open|Close\")"
        n115 = Unbundle By Name(w366) -> ("datos.Ensayo"=w422:T4, "data array"=w409:T4[], "nPuntos"=w406:i32)
        n116 = Unbundle By Name(w366) -> ("Constantes.Ensayo.Vel.min_fluido, m/s"=w365:dbl, "Constantes.Ensayo.Vel_arrastre, m/s"=w364:dbl)
        n117 = Decrement(x=w406) -> (x-1=w425:i32)
        n118 = Rotate 1D Array(1:w409, 2:-1 ("n")) -> (0:w424:T4[])
        n119 = Replace Array Subset(array=w424, new element=w422, index=w425) -> (w407:T4[])
        n120 = for {
          tunnel: [w451] -> w363 mode=indexing
          tunnel: [w450] -> w415 mode=indexing
          tunnel: [w449] -> w416 mode=indexing
          tunnel: [w448] -> w417 mode=indexing
          tunnel: [w447] -> w418 mode=indexing
          tunnel: [w446] -> w419 mode=indexing
          tunnel: [w445] -> w420 mode=indexing
          tunnel: [w444] -> w421 mode=indexing
          tunnel: [w443] -> w410 mode=indexing
          tunnel: [w442] -> w411 mode=indexing
          tunnel: [w441] -> w412 mode=indexing
          tunnel: [w440] -> w413 mode=indexing
          tunnel: [w439] -> w414 mode=indexing
          tunnel: w407 -> [w438] mode=indexing
          tunnel: [w437] -> w382 mode=indexing
          tunnel: [w436] -> w381 mode=indexing
          tunnel: [w435] -> w380 mode=indexing
          tunnel: [w434] -> w379 mode=indexing
          tunnel: [w433] -> w378 mode=indexing
          tunnel: [w432] -> w377 mode=indexing
          tunnel: [w431] -> w376 mode=indexing
          tunnel: [w430] -> w375 mode=indexing
          tunnel: w365 -> [w429]
          tunnel: [w429] -> w361 mode=indexing
          tunnel: [w428] -> w362 mode=indexing
          tunnel: w364 -> [w428]
          n121 = Unbundle By Name(w438) -> ("Tiempo (min)"=w451:dbl, "P116.set.temp, C"=w450:dbl, "P116.temperatura, C"=w449:dbl, "Temp.pt100.1, C"=w448:dbl, "Temp.pt100.2, C"=w447:dbl, "Q.set.caudal, g/s"=w446:dbl, "Q.caudal, g/s"=w445:dbl, "P116.output, W"=w444:dbl, "Humedad.lecho, f1"=w443:dbl, "Agua.evapor, g/s"=w442:dbl, "Q.aire.seco, W"=w441:dbl, "Q.evaporacion, W"=w440:dbl, "Temperatura.ext, C"=w439:dbl, "Temp.pt100.3, C"=w437:dbl, "Temp.pt100.4, C"=w436:dbl, "Temp.termopar.5, C"=w435:dbl, "Temp.termopar.6, C"=w434:dbl, "Humedad.rel.3, f1"=w433:dbl, "Humedad.rel.4, f1"=w432:dbl, "Q.caudal.vol, m3/h"=w431:dbl, "Vel.air.reactor, m/s"=w430:dbl)
        }
        n122 = Bundle(w363, w415) -> (w405:cluster{dbl[], dbl[]})  [unwired: 1 in]
        n123 = Bundle(w363, w416) -> (w404:cluster{dbl[], dbl[]})  [unwired: 1 in]
        n124 = Bundle(w363, w417) -> (w403:cluster{dbl[], dbl[]})  [unwired: 1 in]
        n125 = Bundle(w363, w418) -> (w402:cluster{dbl[], dbl[]})  [unwired: 1 in]
        n126 = Bundle(w363, w419) -> (w401:cluster{dbl[], dbl[]})  [unwired: 1 in]
        n127 = Bundle(w363, w420) -> (w400:cluster{dbl[], dbl[]})  [unwired: 1 in]
        n128 = Bundle(w363, w421) -> (w399:cluster{dbl[], dbl[]})  [unwired: 1 in]
        n129 = Bundle(w363, w410) -> (w398:cluster{dbl[], dbl[]})  [unwired: 1 in]
        n130 = Bundle(w363, w411) -> (w397:cluster{dbl[], dbl[]})  [unwired: 1 in]
        n131 = Bundle(w363, w412) -> (w396:cluster{dbl[], dbl[]})  [unwired: 1 in]
        n132 = Bundle(w363, w413) -> (w395:cluster{dbl[], dbl[]})  [unwired: 1 in]
        n133 = Bundle(w363, w414) -> (w388:cluster{dbl[], dbl[]})  [unwired: 1 in]
        n134 = Bundle(w363, w382) -> (w374:cluster{dbl[], dbl[]})  [unwired: 1 in]
        n135 = Bundle(w363, w381) -> (w373:cluster{dbl[], dbl[]})  [unwired: 1 in]
        n136 = Bundle(w363, w380) -> (w372:cluster{dbl[], dbl[]})  [unwired: 1 in]
        n137 = Bundle(w363, w379) -> (w371:cluster{dbl[], dbl[]})  [unwired: 1 in]
        n138 = Bundle(w363, w378) -> (w370:cluster{dbl[], dbl[]})  [unwired: 1 in]
        n139 = Bundle(w363, w377) -> (w369:cluster{dbl[], dbl[]})  [unwired: 1 in]
        n140 = Bundle(w363, w376) -> (w368:cluster{dbl[], dbl[]})  [unwired: 1 in]
        n141 = Bundle(w363, w375) -> (w367:cluster{dbl[], dbl[]})  [unwired: 1 in]
        n142 = Bundle(w363, w361) -> (w360:cluster{dbl[], dbl[]})  [unwired: 1 in]
        n143 = Bundle(w363, w362) -> (w359:cluster{dbl[], dbl[]})  [unwired: 1 in]
        n144 = Build Array(w398) -> (→"CONCENTRACION HUMEDAD":cluster{dbl[], dbl[]}[])
        n145 = Build Array(w397) -> (→"AGUA EVAPORADA AL AIRE":cluster{dbl[], dbl[]}[])
